vi "ShopInfo.vi"() -> (0 "商店信息":T1)   [LabVIEW 2013, in "ShopBase.lvclass"]
uses:
  ShopBase.lvclass
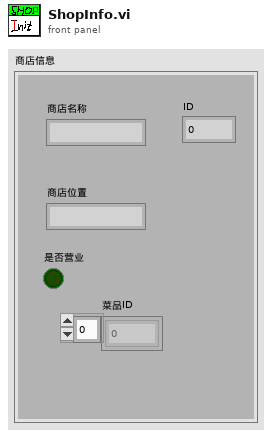
[diagram p1: front panel]
types:
  T1 = cluster{"ID":dbl, "商店名称":string, "商店位置":string, "是否营业":bool, "菜品ID":dbl[]}
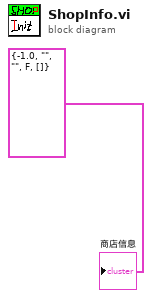
[diagram p0: block diagram]
diagram:
  "商店信息" <- T1 {"ID"=-1.0, "商店名称"="", "商店位置"="", "是否营业"=FALSE, "菜品ID"=[]} ("商店信息 2")
